vi "Setup Hardware.vi"(8 "error in (no error)":errorcluster, 11 "Global Ctrls For Saving":T1={"Time Stamp"={"date string"="", "time string"=""}, "Exp Params"={"Experiment Type"="Time Series", "Experiment Name"="Experiment_1", "ExpPath"=path "D:/Data", "Save As"="TIFF", "TSFrames"=1000, "TSfps"=1.0, "Streaming"=TRUE, "tdms ref"=refnum, "frame #"=0, "Full Path"=path "", "PeakOnQueue"=FALSE}, "Ventus Controls"={"Ventus Power"=0.0, "Open Serial"=FALSE, "VISA Refnum"="ASRL5::INSTR"}, "Camera Controls"={"Exposure Time (ms)"=27, "cam0 Session"="cam0", "Camera ROI"={"Width"=0, "Height"=0, "Offset X"=0, "Offset Y"=0}, "Command"=""}, "Spot Params"=[{"Intensity"=0.0, "Vortex"=0.0, "Phase"=0.0, "X"=0.0, "Y"=0.0, "Z"=0.0}], "SLM Parameters"={"Width"=0.0, "Height"=0.0, "Board ID"=0, "Centre Y"=0.0, "Centre X"=0.0}} {"Spot Params"."Z" format="%_4g"; "Spot Params"."Y" format="%_4g"; "Spot Params"."X" format="%_4g"; "Spot Params"."Phase" format="%_4g"; "Spot Params"."Intensity" format="%_4g"; "Camera Controls"."Camera ROI"."Offset Y" max=2046 step=2; "Camera Controls"."Camera ROI"."Offset X" max=2044 step=4; "Camera Controls"."Camera ROI"."Height" min=2 max=2048 step=2; "Camera Controls"."Camera ROI"."Width" min=4 max=2048 step=4; "Camera Controls"."Exposure Time (ms)" min=27 max=500 step=1 scale=27.0..500.0; "SLM Parameters"."Centre X" format="%.3g"; "SLM Parameters"."Centre Y" format="%.3g"; "Ventus Controls"."Ventus Power" min=0.0 max=100.0 step=0.1 scale=0.0..100.0; "Exp Params"."TSFrames" min=1 step=1; "Exp Params"."TSfps" min=0.001 max=90.0 step=0.001 format="%_4g"}) -> (0 "error out":errorcluster, 3 "Global Ctrls For Saving out":T1={"Time Stamp"={"date string"="", "time string"=""}, "Exp Params"={"Experiment Type"="Time Series", "Experiment Name"="Experiment_1", "ExpPath"=path "D:/Data", "Save As"="TIFF", "TSFrames"=1000, "TSfps"=1.0, "Streaming"=TRUE, "tdms ref"=refnum, "frame #"=0, "Full Path"=path "", "PeakOnQueue"=FALSE}, "Ventus Controls"={"Ventus Power"=0.0, "Open Serial"=FALSE, "VISA Refnum"="ASRL5::INSTR"}, "Camera Controls"={"Exposure Time (ms)"=27, "cam0 Session"="cam0", "Camera ROI"={"Width"=0, "Height"=0, "Offset X"=0, "Offset Y"=0}, "Command"=""}, "Spot Params"=[{"Intensity"=0.0, "Vortex"=0.0, "Phase"=0.0, "X"=0.0, "Y"=0.0, "Z"=0.0}], "SLM Parameters"={"Width"=0.0, "Height"=0.0, "Board ID"=0, "Centre Y"=0.0, "Centre X"=0.0}} {"Spot Params"."Z" format="%_4g"; "Spot Params"."Y" format="%_4g"; "Spot Params"."X" format="%_4g"; "Spot Params"."Phase" format="%_4g"; "Spot Params"."Intensity" format="%_4g"; "Camera Controls"."Camera ROI"."Offset Y" max=2046 step=2; "Camera Controls"."Camera ROI"."Offset X" max=2044 step=4; "Camera Controls"."Camera ROI"."Height" min=2 max=2048 step=2; "Camera Controls"."Camera ROI"."Width" min=4 max=2048 step=4; "Camera Controls"."Exposure Time (ms)" min=27 max=500 step=1 scale=27.0..500.0; "SLM Parameters"."Centre X" format="%.3g"; "SLM Parameters"."Centre Y" format="%.3g"; "Ventus Controls"."Ventus Power" min=0.0 max=100.0 step=0.1 scale=0.0..100.0; "Exp Params"."TSFrames" min=1 step=1; "Exp Params"."TSfps" min=0.001 max=90.0 step=0.001 format="%_4g"}, 4 "Camera Connected":bool, 6 "Trapping Laser Connected":bool)   [LabVIEW 2020]
uses:
  _controls/PCIe SLM params.ctl
  <vilib>/userDefined/High Color/IMAQdx.ctl
  _controls/xiCam.ctl
  _controls/Trapping Laser Control.ctl
  _controls/Exp Params.ctl
  _controls/Spot Params.ctl
  _controls/Global Ctrls For Saving.ctl
panel:
  out "VISA Refnum out":refnum<visa-resource-name>
  out "Errors":string
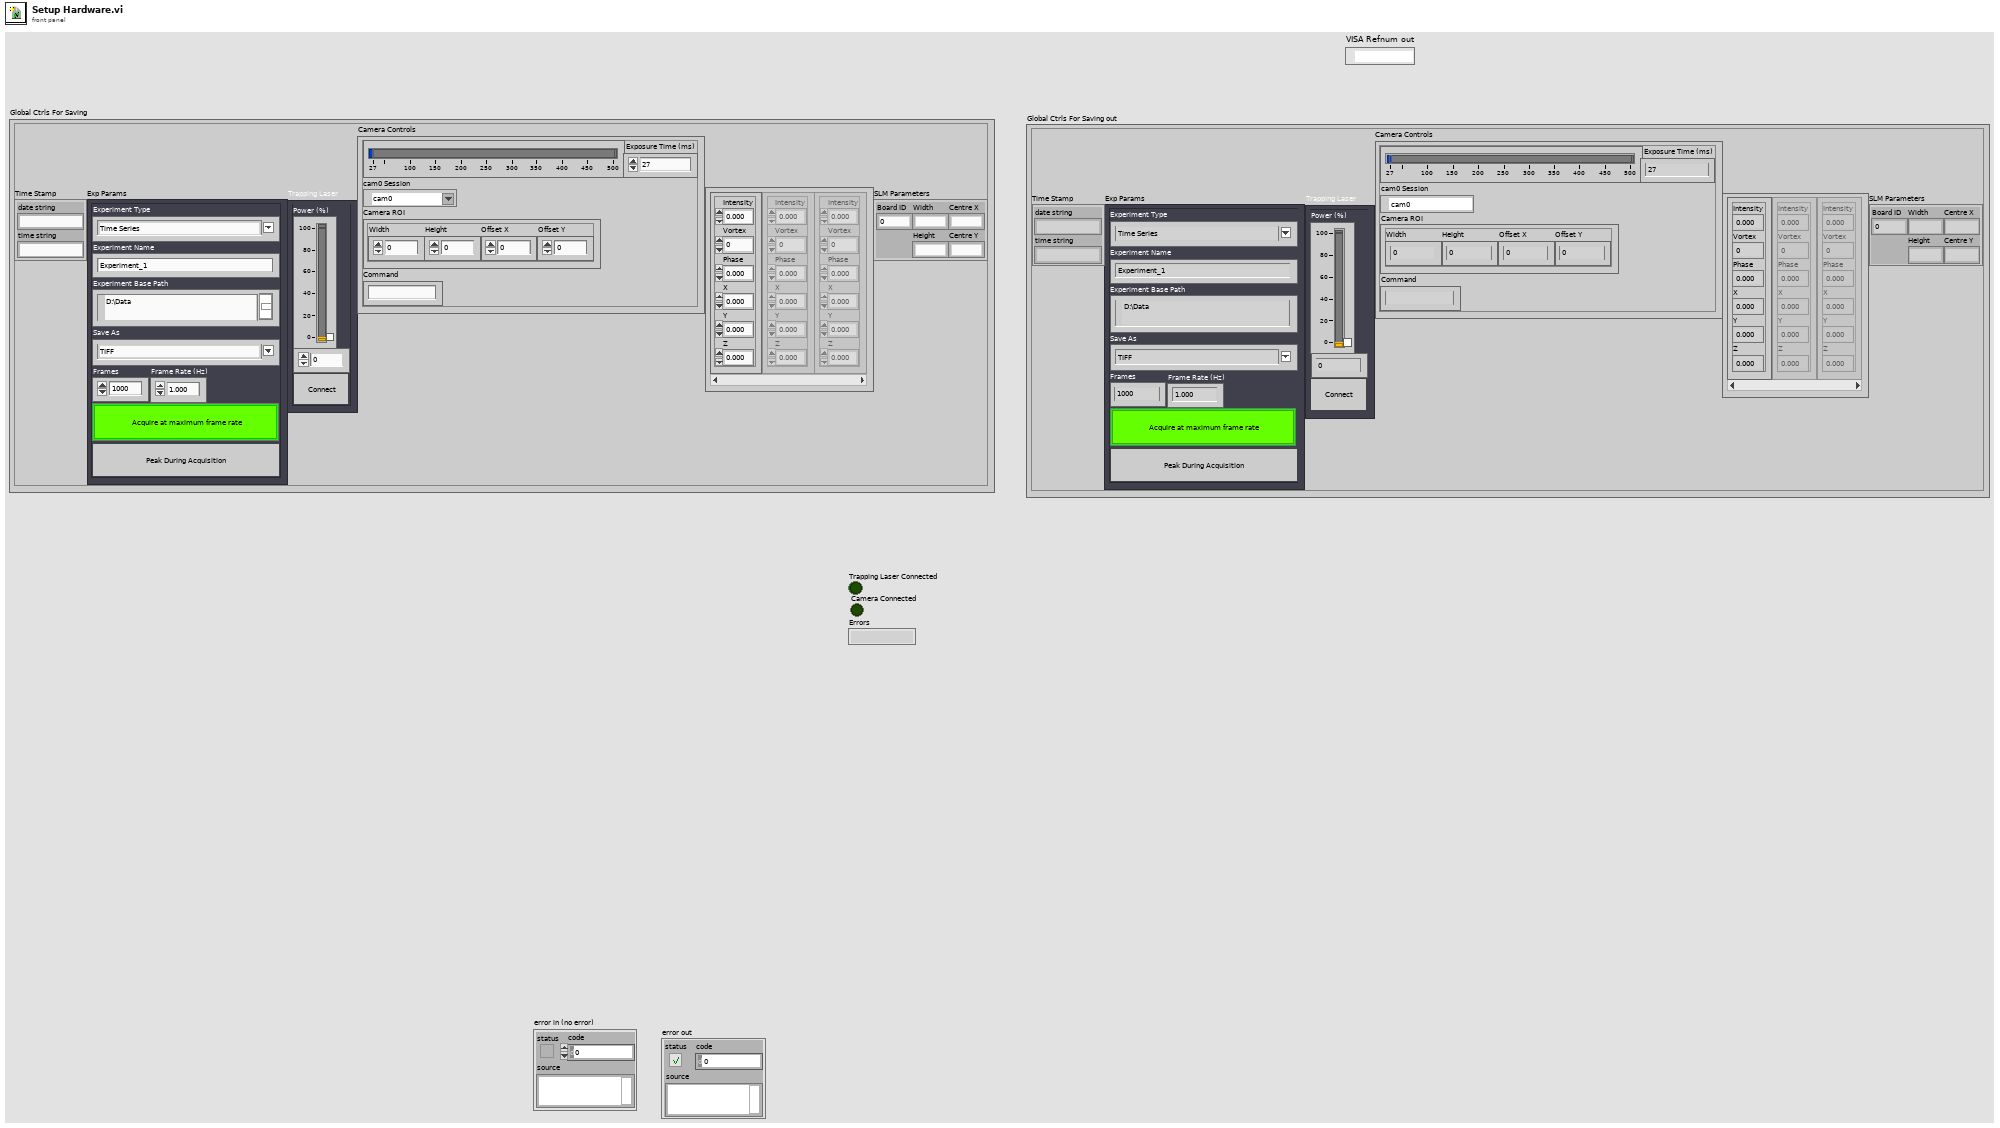
[diagram p1: front panel]
types:
  T1 = typedef "Global Ctrls For Saving.ctl" = cluster{"Time Stamp":cluster{"date string":string, "time string":string}, "Exp Params":T2, "Ventus Controls":T3, "Camera Controls":T4, "Spot Params":T6, "SLM Parameters":T7}
  T2 = typedef "Exp Params.ctl" = cluster{"Experiment Type":string, "Experiment Name":string, "ExpPath":path, "Save As":string, "TSFrames":i32, "TSfps":dbl, "Streaming":bool, "tdms ref":refnum<k34>, "frame #":i64, "Full Path":path, "PeakOnQueue":bool}
  T3 = typedef "Trapping Laser Control.ctl" = cluster{"Ventus Power":dbl, "Open Serial":bool, "VISA Refnum":refnum<visa-resource-name>}
  T4 = typedef "xiCam.ctl" = cluster{"Exposure Time (ms)":u32, "cam0 Session":T5, "Camera ROI":cluster{"Width":u32, "Height":u32, "Offset X":u32, "Offset Y":u32}, "Command":string}
  T5 = typedef "IMAQdx.ctl" = refnum<k21>
  T6 = typedef "Spot Params.ctl" = cluster{"Intensity":dbl, "Vortex":dbl, "Phase":dbl, "X":dbl, "Y":dbl, "Z":dbl}[]
  T7 = typedef "PCIe SLM params.ctl" = cluster{"Width":dbl, "Height":dbl, "Board ID":i32, "Centre Y":dbl, "Centre X":dbl}
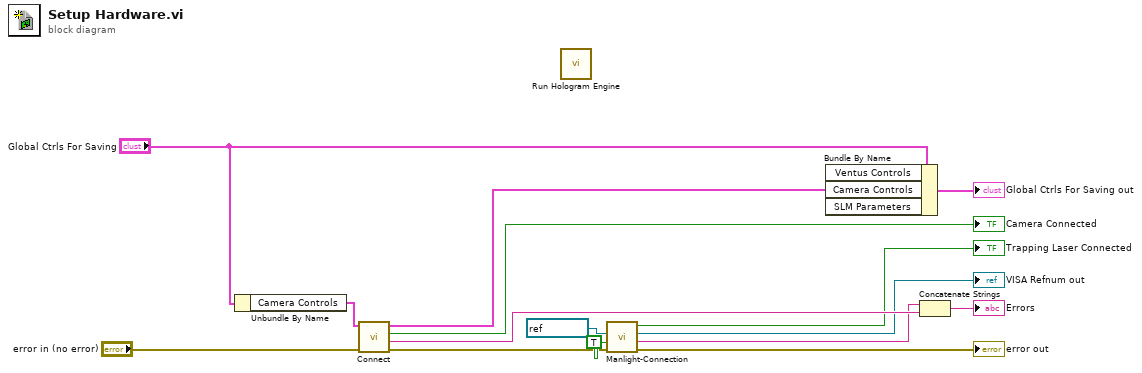
[diagram p0: block diagram]
diagram:
  n1 = Unbundle By Name("Global Ctrls For Saving") -> ("Camera Controls"=w13:T4)
  n2 = call "Connect.vi"("error in (no error)"="error in (no error)", "Camera Controls in"=w13) -> ("error out"=w6:errorcluster, "String"=w15:string, "Camera Connected"=→"Camera Connected":bool, "Camera Controls out"=w10:T4)  [unwired: 6 in]
  n3 = call "Run Hologram Engine.vi"() -> ()  [unwired: 11 in, 1 out]
  n4 = call "Manlight-Connection.vi"("error in"=w6, "Connect?"=TRUE, "VISA Refnum in"=refnum<visa-resource-name> "COM4") -> ("error out"=→"error out":errorcluster, "Status"=w4:string, "VISA Refnum out"=→"VISA Refnum out":refnum<visa-resource-name>, "Manlight Laser Connected"=→"Trapping Laser Connected":bool)  [unwired: 1 in]
  n5 = Bundle By Name(cluster="Global Ctrls For Saving", "Camera Controls"=w10) -> (→"Global Ctrls For Saving out":T1)  [unwired: 2 in]
  n6 = Concatenate Strings(w4, w15) -> (→"Errors":string)
